vi "Cycle.vi"(8 "error in (no error)":errorcluster, 11 "BehaviorClassification In":refnum<class "ClassDiscrimination.lvclass">) -> (0 "error out":errorcluster, 3 "BehaviorClassification Out":refnum<class "ClassDiscrimination.lvclass">)   [LabVIEW 2014, in "ClassDiscrimination.lvclass"]
uses:
  ClassDiscrimination.lvclass
  ClassDiscrimination.lvclass/ClassDiscrimination.ctl
  Trial Based Experiment Statechart/MatlabExperiment/MatlabExperiment.lvclass
panel:
  in  "Punish time":dbl=1000.0
  in  "Eye Params":dbl[](array[numeric])
  out "XY Graph":cluster{dbl[], dbl[]}(graph)
  in  "RewardAmount":dbl=50.0
  in  "FixationRadius":dbl=50.0
  out "Timeouts":T1={"Intertrial"=1000.0, "AcquireFixation"=1000.0, "HoldFixation"=300.0, "DelayPeriod"=1000.0, "ResponsePeriod"=1000.0}
  out "ExperimentStats":T2
  out "Cycles":dbl
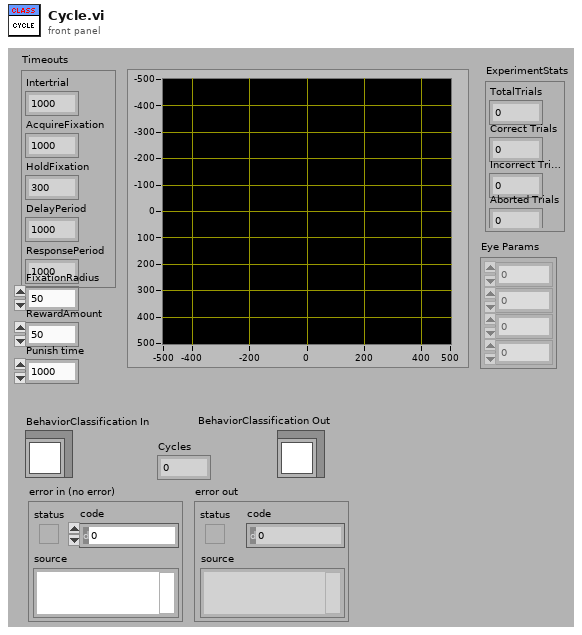
[diagram p1: front panel]
types:
  T1 = cluster{"Intertrial":dbl, "AcquireFixation":dbl, "HoldFixation":dbl, "DelayPeriod":dbl, "ResponsePeriod":dbl}
  T2 = cluster{"TotalTrials":dbl, "Correct Trials":dbl, "Incorrect Trials":dbl, "Aborted Trials":dbl}
  T3 = cluster{"TotalTrials":u32, "Correct Trials":u32, "Incorrect Trials":u32, "Aborted Trials":u32}
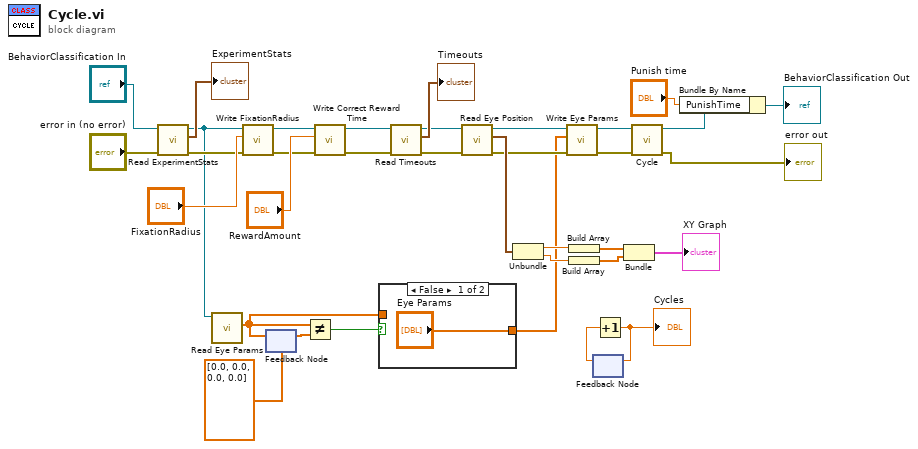
[diagram p0: block diagram]
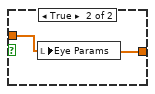
[diagram p2: hidden frame]
diagram:
  n1 = call-dynamic "Read ExperimentStats.vi"("error in (no error)"="error in (no error)", "TrialBasedExperiment in"="BehaviorClassification In") -> ("error out"=w25:errorcluster, "ExperimentStats"=→"ExperimentStats":T3, "TrialBasedExperiment out"=w9:refnum<class "ClassDiscrimination.lvclass">)  [unwired: 7 in]
  n2 = call-dynamic "Read Eye Params.vi"("TrialBasedExperiment in"=w9) -> ("Eye Params"=w6:dbl[])  [unwired: 8 in, 2 out]
  n3 = call-dynamic "Write FixationRadius.vi"("error in (no error)"=w25, "FixationRadius"="FixationRadius", "MatlabExperiment in"=w9) -> ("error out"=w24:errorcluster, "MatlabExperiment out"=w27:refnum<class "ClassDiscrimination.lvclass">)  [unwired: 7 in]
  n4 = feedback-in #1(w6) -> ()
  n5 = feedback #1(dbl[] [0.0, 0.0, 0.0, 0.0] ("Eye Params")) -> (w8:dbl[])
  n6 = Not Equal?(x=w6, y=w8) -> (x != y?=w7:bool)
  n7 = call-dynamic "Write Correct Reward Time.vi"("error in (no error)"=w24, "Correct Reward Time"="RewardAmount", "MatlabExperiment in"=w27) -> ("error out"=w23:errorcluster, "MatlabExperiment out"=w26:refnum<class "ClassDiscrimination.lvclass">)  [unwired: 7 in]
  n8 = case shown="False" w7 {
    tunnel: w6 -> [_ w37]
    tunnel: ["Eye Params" w37] -> w5
    frame False {
    }
    frame True {
      n9 = local write "Eye Params"(w37) -> ()
    }
  }
  n10 = call-dynamic "Read Timeouts.vi"("error in (no error)"=w23, "TrialBasedExperiment in"=w26) -> ("error out"=w15:errorcluster, "Timeouts"=→"Timeouts":T1, "TrialBasedExperiment out"=w16:refnum<class "ClassDiscrimination.lvclass">)  [unwired: 7 in]
  n11 = call-dynamic "Read Eye Position.vi"("error in (no error)"=w15, "TrialBasedExperiment in"=w16) -> ("error out"=w13:errorcluster, "Eye Position"=w22:cluster{"Horizontal":dbl, "Vertical":dbl}, "TrialBasedExperiment out"=w14:refnum<class "ClassDiscrimination.lvclass">)  [unwired: 7 in]
  n12 = Unbundle(w22) -> ("Horizontal"=w21:dbl, "Vertical"=w20:dbl)
  n13 = call-dynamic "Write Eye Params.vi"("error in (no error)"=w13, "Eye Params"=w5, "TrialBasedExperiment in"=w14) -> ("error out"=w11:errorcluster, "TrialBasedExperiment out"=w12:refnum<class "ClassDiscrimination.lvclass">)  [unwired: 7 in]
  n14 = Build Array(w21) -> (w19:dbl[])
  n15 = Build Array(w20) -> (w18:dbl[])
  n16 = feedback #2() -> (w34:dbl)  [unwired: 1 in]
  n17 = Increment(x=w34) -> (x+1=w35:dbl)
  "Cycles" <- w35
  n18 = feedback-in #2(w35) -> ()
  n19 = Bundle(w19, w18) -> (→"XY Graph":cluster{dbl[], dbl[]})  [unwired: 1 in]
  n20 = call-parent "Cycle.vi"("error in (no error)"=w11, "MatlabExperiment In"=w12) -> ("error out"=→"error out":errorcluster, "MatlabExperiment Out"=w3:refnum<class "ClassDiscrimination.lvclass">)  [unwired: 8 in]
  n21 = Bundle By Name(cluster=w3, "PunishTime"="Punish time") -> (→"BehaviorClassification Out":refnum<class "ClassDiscrimination.lvclass">)
